vi "get_refnum.vi"(11 "MultipartForm":refnum<class "MultipartForm.lvclass">) -> (2 "ref":u64)   [LabVIEW 2020, in "reqwest.lvlib" / "MultipartForm.lvclass"]
uses:
  MultipartForm.lvclass
  MultipartForm.lvclass/MultipartForm.ctl
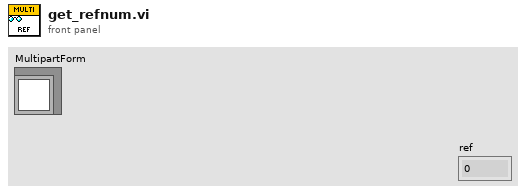
[diagram p1: front panel]
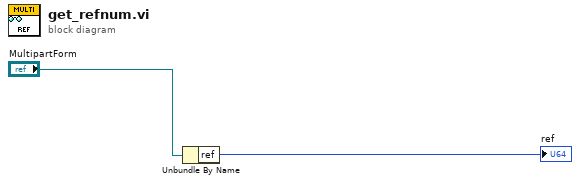
[diagram p0: block diagram]
diagram:
  n1 = Unbundle By Name("MultipartForm") -> ("ref"=→"ref":u64)
